vi "Get Control Data Type.vi"(4 "error in (no error)":errorcluster, 7 "Control Refnum in":refnum<vi>) -> (0 "error out":errorcluster, 2 "Control's Data Type":variant, 3 "Control Refnum out":refnum<vi>)   [LabVIEW 2020]
doc: "Given a control refnum, this VI returns the data type of that control as a LabVIEW Variant."
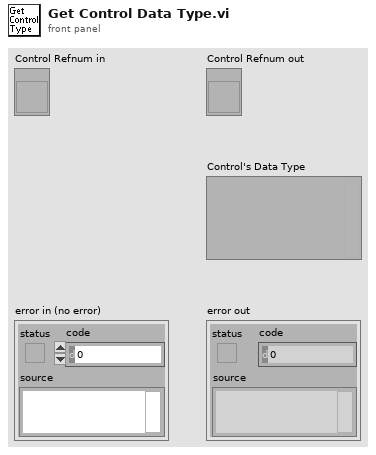
[diagram p1: front panel]
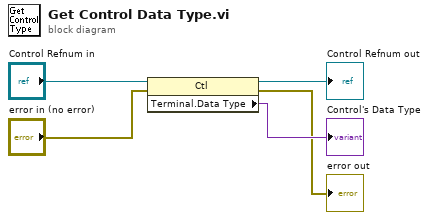
[diagram p0: block diagram]
diagram:
  n1 = property class="Ctl"(reference="Control Refnum in", error in="error in (no error)") -> (reference out=→"Control Refnum out":refnum<vi>, error out=→"error out":errorcluster, "Terminal.Data Type"=→"Control's Data Type":variant)
